vi "Count number of balls shot.vi"(9 "Number of balls wait for":dbl, 10 "Current Threshold":dbl format="%#_13g", 11 "PhoenixMotorControlDevRef":T1) -> (3 "Done?":bool)   [LabVIEW 2019]
uses:
  Shoot Global.vi
  <vilib>/Rock Robotics/WPI/ThirdParty/Phoenix-LabVIEW/Motor Controller/Get/CTRE_Phoenix_MotorController_GetSupplyAndStatorCurrent_Enhanced.vi
  <vilib>/Rock Robotics/SystemInterfaces/DIO/FPGA_DIOPWMChannel.ctl
  <vilib>/Rock Robotics/WPI/PWM/WPI_PWMDeadband.ctl
  <vilib>/Rock Robotics/WPI/MotorControl/WPI_MotorControlType.ctl
  <vilib>/Rock Robotics/SystemInterfaces/DIO/FPGA_DIOChannel.ctl
  <vilib>/Rock Robotics/WPI/MotorControl/WPI_MotorControlDeviceRef.ctl
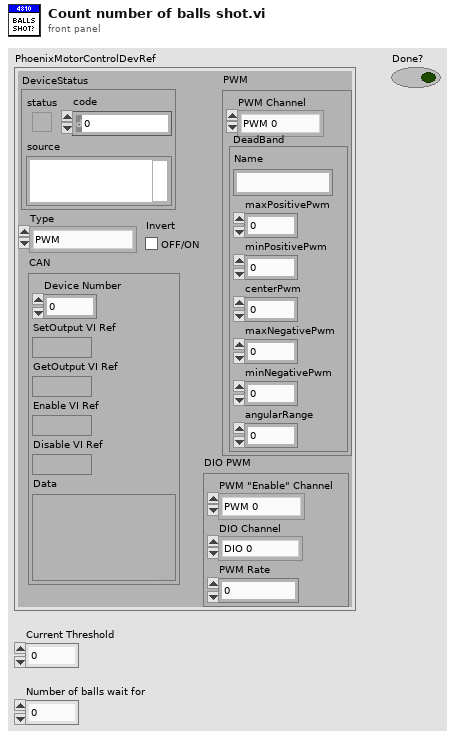
[diagram p1: front panel]
types:
  T1 = typedef "WPI_MotorControlDeviceRef.ctl" = cluster{"DeviceStatus":errorcluster, "Type":T2, "PWM":cluster{"PWM Channel":T3, "DeadBand":T4}, "CAN":cluster{"Device Number":u8, "SetOutput VI Ref":variant, "GetOutput VI Ref":variant, "Enable VI Ref":variant, "Disable VI Ref":variant, "Data":variant}, "Invert":bool, "DIO PWM":cluster{"PWM \"Enable\" Channel":T3, "DIOChannel":T5, "PWM Rate":dbl}}
  T2 = typedef "WPI_MotorControlType.ctl" = enum16{"PWM", "CAN", "DIO PWM"}
  T3 = typedef "FPGA_DIOPWMChannel.ctl" = enum8{"PWM 0", "PWM 1", "PWM 2", "PWM 3", "PWM 4", "PWM 5", "PWM 6", "PWM 7", "PWM 8", "PWM 9", "PWM MXP 0", "PWM MXP 1", "PWM MXP 2", "PWM MXP 3", "PWM MXP 4", "PWM MXP 5", "PWM MXP 6", "PWM MXP 7", "PWM MXP 8", "PWM MXP 9", "Invalid"}
  T4 = typedef "WPI_PWMDeadband.ctl" = cluster{"Name":string, "maxPositivePwm":i32, "minPositivePwm":i32, "centerPwm":i32, "maxNegativePwm":i32, "minNegativePwm":i32, "angularRange":u16}
  T5 = typedef "FPGA_DIOChannel.ctl" = enum8{"DIO 0", "DIO 1", "DIO 2", "DIO 3", "DIO 4", "DIO 5", "DIO 6", "DIO 7", "DIO 8", "DIO 9", "DIO MXP 0", "DIO MXP 1", "DIO MXP 2", "DIO MXP 3", "DIO MXP 4", "DIO MXP 5", "DIO MXP 6", "DIO MXP 7", "DIO MXP 8", "DIO MXP 9", "DIO MXP 10", "DIO MXP 11", "DIO MXP 12", "DIO MXP 13", "DIO MXP 14", "DIO MXP 15", "SPI Port CS1", "SPI Port CS2", "SPI Port CS3", "SPI Port MISO", "SPI Port MOSI", "Invalid"}
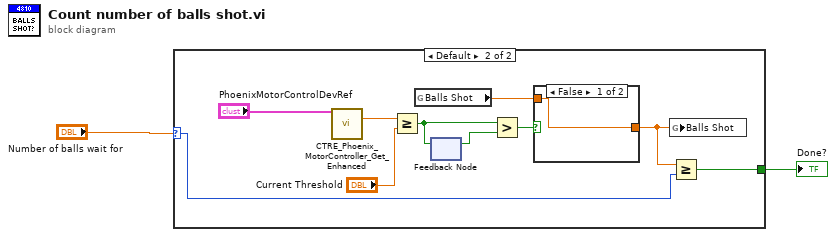
[diagram p0: block diagram]
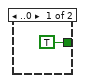
[diagram p2: hidden frame]
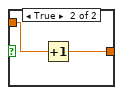
[diagram p3: hidden frame]
diagram:
  n1 = case shown="Default" "Number of balls wait for" {
    selector: "Number of balls wait for" -> [_ w4]
    tunnel: [TRUE w13] -> w2
    frame ..0 {
    }
    frame Default {
      n2 = call-poly <vilib>:"CTRE_Phoenix_MotorController_Get_Enhanced.vi"("PhoenixMotorControlDevRef"="PhoenixMotorControlDevRef") -> ("Supply Current"=w7:dbl)  [unwired: 11 in, 3 out]
      n3 = Greater Or Equal?(x=w7, y="Current Threshold") -> (x >= y?=w9:bool)
      n4 = global read "Shoot Global.vi" "Balls Shot"() -> (w11:dbl)
      n5 = feedback #1() -> (w8:bool)  [unwired: 1 in]
      n6 = feedback-in #1(w9) -> ()
      n7 = Greater?(x=w9, y=w8) -> (0:w10:bool)
      n8 = case shown="False" w10 {
        tunnel: [w14 w16] -> w12
        tunnel: w11 -> [w14 w15]
        frame False {
        }
        frame True {
          n9 = Increment(x=w15) -> (x+1=w16:dbl)
        }
      }
      n10 = global write "Shoot Global.vi" "Balls Shot"(w12) -> ()
      n11 = Greater Or Equal?(x=w12, y=w4) -> (x >= y?=w13:bool)
    }
  }
  "Done?" <- w2
